vi "TorqueData.vi"() -> ()   [LabVIEW 2020]
panel:
  out "Numeric Indicator":dbl
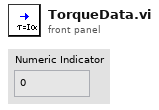
[diagram p1: front panel]
diagram:
